vi "全局变量.vi"() -> ()   [LabVIEW 2014]
panel:
  out "前截图":bool
  out "前摄像":bool
  out "后截图":bool
  out "主截图":bool
  out "后录像":bool
  out "主录像":bool
  out "焦点":u8
  out "焦距":u8
  out "姿态":cluster{"PITCH":dbl, "BANK":dbl, "HEANDING":dbl}
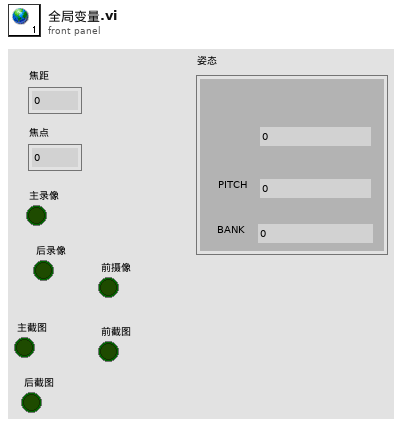
[diagram p1: front panel]
diagram:
